vi "WS1021 ADI OFFSET CAL.vi"(6 "DUT Mask Mode (All)":T1=enum."All", 7 "FPGA":T2, 8 "Error In":errorcluster) -> (0 "Error Out":errorcluster)   [LabVIEW 2017]
uses:
  WS_VCAP Driver 1_49/Source/WSVCAP Shell/Type Defs/WSVCAP SHL FPGA Enum.ctl
  WS_VCAP Driver 1_49/Source/WSVCAP Shell/Type Defs/WSVCAP SHL I2C DUT Mask Mode Enum.ctl
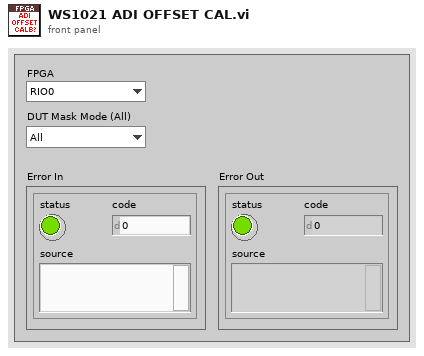
[diagram p1: front panel]
types:
  T1 = typedef "WSVCAP SHL I2C DUT Mask Mode Enum.ctl" = enum16{"Custom", "All"}
  T2 = typedef "WSVCAP SHL FPGA Enum.ctl" = enum16{"RIO0", "RIO1"}
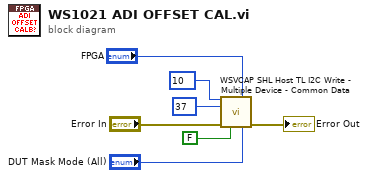
[diagram p0: block diagram]
diagram:
  n1 = call "WSVCAP SHL Host TL I2C Write - Multiple Device - Common Data.vi"("Sub Address"=u8 10, "FPGA"="FPGA", "Data Out [U8]"=u8 37 ("Sub Address"), "error in"="Error In", "Log (T)"=FALSE, "DUT Mask Mode (All)"="DUT Mask Mode (All)") -> ("error out"=→"Error Out":errorcluster)  [unwired: 9 in]
